vi "Global Variables.vi"() -> ()   [LabVIEW 2013]
panel:
  in  "Reset Tacs?":bool
  in  "J2 Xbox Back":bool
  in  "J2 Xbox Start":bool
  in  "J2 Xbox RB":bool
  in  "Fire":bool
  in  "Pivots Enabled?":bool=TRUE
  in  "J1 Xbox B":bool
  in  "J1 Xbox Y":bool
  in  "J1 Xbox X":bool
  in  "J1 Xbox Select":bool
  in  "J1 Xbox LB":bool
  in  "J1 Xbox RB":bool
  in  "J1 Xbox A":bool
  in  "Calibration BR":dbl
  in  "Calibration BL":dbl
  in  "Calibration FR":dbl
  in  "Calibration FL":dbl
  in  "Rotational Motor BR":dbl
  in  "Rotational Motor BL":dbl
  in  "Rotational Motor FR":dbl
  in  "Rotational Motor FL":dbl
  in  "Drive Motor BR":dbl
  in  "Drive Motor BL":dbl
  in  "Drive Motor FR":dbl
  in  "Drive Motor FL":dbl
  # "Steering"
  # "Drive"
  # "Calibration"
  # "Buttons"
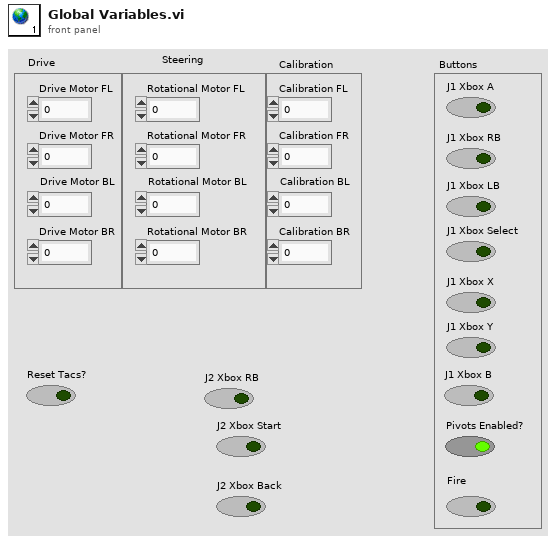
[diagram p1: front panel]
diagram:
